vi "rszvl_core_global.vi"() -> ()   [LabVIEW 2014] (continued)
, "Flags"={"OPC Wait"=FALSE, "Dont check status"=FALSE, "*WAI"=FALSE}, "Check Status Callback"=""}, {"Level"=3, "Descriptive Name"="Delta Marker Mode", "Class Only"=FALSE, "Data Type"=0, "Access"=2, "Identifier"="RSZVL_ATTR_REFERENCE_MARKER_MODE", "Range Table"="rszvl_rngAbsRel", "Command"="CALC:DELT{DeltaMarker}:MODE", "Read Callback"="", "Write Callback"="", "Range Callback"="", "Check Callback"="", "Rngtable Callback"="", "Coerce Callback"="", "User Callback"="", "Supported Models"="", "Instrument Options"="", "Repeated Capabilities"="", "Restricted Repeated Capabilities"="", "Help"="This attribute switches between relative and absolute frequency input of the delta marker (or time with span = 0). It affects all delta markers.\nRepeated capabilitiy Delta Marker are used to prevent switching On Delta Marker 1, if the user uses Delta Marker 2.\n\nAvailable Repeated Capabilities:\nDeltaMarker: DM1,DM2,DM3,DM4\r\n\nRemote-control command(s):\nCALCulate<1|2>:DELTamarker<1 to 4>:MODE ABSolute | RELative", "Flags"={"OPC Wait"=FALSE, "Dont check status"=FALSE, "*WAI"=FALSE}, "Check Status Callback"=""}, {"Level"=3, "Descriptive Name"="Delta Marker Position", "Class Only"=FALSE, "Data Type"=1, "Access"=2, "Identifier"="RSZVL_ATTR_REFERENCE_MARKER_POSITION", "Range Table"="", "Command"="CALC:DELT{DeltaMarker}:X", "Read Callback"="", "Write Callback"="", "Range Callback"="", "Check Callback"="", "Rngtable Callback"="", "Coerce Callback"="", "User Callback"="", "Supported Models"="", "Instrument Options"="", "Repeated Capabilities"="", "Restricted Repeated Capabilities"="", "Help"="This attribute positions the selected delta marker to the indicated frequency (span > 0), time (span = 0) or level (APD measurement = ON or CCDFmeasurement = ON). The input is in absolute values or relative to marker 1 depending on the attribute RSZVL_ATTR_REFERENCE_MARKER_MODE. If Reference Fixed measurement (CALCulate:DELTamarker:FUNCtion:FIXed:STATe ON) is active, relative values refer to the reference position are entered. The query always returns absolute values.\n\nAvailable Repeated Capabilities:\nDeltaMarker: DM1,DM2,DM3,DM4\r\n\nRemote-control command(s):\nCALCulate<1|2>:DELTamarker<1 to 4>:X", "Flags"={"OPC Wait"=FALSE, "Dont check status"=FALSE, "*WAI"=FALSE}, "Check Status Callback"=""}, {"Level"=3, "Descriptive Name"="Delta Marker Relative Position", "Class Only"=FALSE, "Data Type"=1, "Access"=0, "Identifier"="RSZVL_ATTR_REFERENCE_MARKER_REL_POSITION", "Range Table"="", "Command"="CALC:DELT{DeltaMarker}:X:REL?", "Read Callback"="", "Write Callback"="", "Range Callback"="", "Check Callback"="", "Rngtable Callback"="", "Coerce Callback"="", "User Callback"="", "Supported Models"="", "Instrument Options"="", "Repeated Capabilities"="", "Restricted Repeated Capabilities"="", "Help"="This attribute queries the frequency (span > 0) or time (span = 0) of the selected delta marker relative to marker 1 or to the reference position ( for CALCulate:DELTamarker:FUNCtion:FIXed:STATe ON). The attribute activates the corresponding delta marker, if necessary.\n\nAvailable Repeated Capabilities:\nDeltaMarker: DM1,DM2,DM3,DM4\r\n\nRemote-control command(s):\nCALCulate<1|2>:DELTamarker<1 to 4>:X:RELative?", "Flags"={"OPC Wait"=FALSE, "Dont check status"=FALSE, "*WAI"=FALSE}, "Check Status Callback"=""}, {"Level"=3, "Descriptive Name"="Delta Marker Amplitude", "Class Only"=FALSE, "Data Type"=1, "Access"=0, "Identifier"="RSZVL_ATTR_REFERENCE_MARKER_AMPLITUDE", "Range Table"="", "Command"="CALC:DELT{DeltaMarker}:Y?", "Read Callback"="", "Write Callback"="", "Range Callback"="", "Check Callback"="", "Rngtable Callback"="", "Coerce Callback"="", "User Callback"="", "Supported Models"="", "Instrument Options"="", "Repeated Capabilities"="", "Restricted Repeated Capabilities"="", "Help"="This attribute queries the measured value of the selected delta marker. The corresponding delta marker will be activated, if necessary. The output is always a relative value referred to marker 1 or to the reference position (reference fixed active).\n\nAvailable Repeated Capabilities:\nDeltaMarker: DM1,DM2,DM3,DM4\r\n\nRemote-control command(s):\nCALCulate<1|2>:DELTamarker<1 to 4>:Y?", "Flags"={"OPC Wait"=FALSE, "Dont check status"=FALSE, "*WAI"=FALSE}, "Check Status Callback"=""}, {"Level"=3, "Descriptive Name"="Delta Marker Assign Trace", "Class Only"=FALSE, "Data Type"=0, "Access"=2, "Identifier"="RSZVL_ATTR_REFERENCE_MARKER_TRACE", "Range Table"="rszvl_rngTrace", "Command"="CALC:DELT{DeltaMarker}:TRAC", "Read Callback"="", "Write Callback"="", "Range Callback"="", "Check Callback"="", "Rngtable Callback"="", "Coerce Callback"="", "User Callback"="", "Supported Models"="", "Instrument Options"="", "Repeated Capabilities"="", "Restricted Repeated Capabilities"="", "Help"="This attribute assigns the selected delta marker to the indicated measurement curve. The selected measurement curve must be active, i.e. its state must be different from BLANK.\n\nAvailable Repeated Capabilities:\nDeltaMarker: DM1,DM2,DM3,DM4\r\n\nRemote-control command(s):\nCALCulate<1|2>:DELTamarker<1 to 4>:TRACe", "Flags"={"OPC Wait"=FALSE, "Dont check status"=FALSE, "*WAI"=FALSE}, "Check Status Callback"=""}, {"Level"=3, "Descriptive Name"="Delta Marker All Off", "Class Only"=FALSE, "Data Type"=4, "Access"=1, "Identifier"="RSZVL_ATTR_REFERENCE_MARKER_AOFF", "Range Table"="", "Command"="CALC:DELT:AOFF", "Read Callback"="", "Write Callback"="", "Range Callback"="", "Check Callback"="", "Rngtable Callback"="", "Coerce Callback"="", "User Callback"="", "Supported Models"="", "Instrument Options"="", "Repeated Capabilities"="", "Restricted Repeated Capabilities"="", "Help"="This attribute switches off all active delta markers (screen A or screen B).\n\nAvailable Repeated Capabilities:\nNone\n\nRemote-control command(s):\nCALCulate<1|2>:DELTamarker<1 to 4>:AOFF", "Flags"={"OPC Wait"=FALSE, "Dont check status"=FALSE, "*WAI"=FALSE}, "Check Status Callback"=""}, {"Level"=2, "Descriptive Name"="Delta Marker Search", "Class Only"=TRUE, "Data Type"=0, "Access"=0, "Identifier"="", "Range Table"="", "Command"="", "Read Callback"="", "Write Callback"="", "Range Callback"="", "Check Callback"="", "Rngtable Callback"="", "Coerce Callback"="", "User Callback"="", "Supported Models"="", "Instrument Options"="", "Repeated Capabilities"="", "Restricted Repeated Capabilities"="", "Help"="Delta marker search.\n\n(1) Delta Marker Peak:\nThis attribute positions the delta marker to the current maximum value on the measured curve. If necessary, the corresponding delta marker will be activated first.\n\n(2) Delta Marker Peak Next:\nThis attribute positions the delta marker to the next smaller maximum value on the measured curve. The corresponding delta marker will be activated first, if necessary.\n\n(3) Delta Marker Peak Next Right:\nThis attribute positions the delta marker to the next smaller maximum value to the right of the current value (i.e. ascending X values). The corresponding delta marker is activated first, if necessary.\n\n(4) Delta Marker Peak Next Left:\nThis attribute positions the delta marker to the next smaller maximum value to the left of the current value (i.e. descending X values). The corresponding delta marker will be activated first, if necessary.\n\n(5) Delta Marker Minimum:\nThis attribute positions the delta marker to the current minimum value on the measured crve. The corresponding delta marker will be activated first, if necessary.\n\n(6) Delta Marker Minimum Next:\nThis attribute positions the delta marker to the next higher minimum value of the measured curve. The corresponding delta marker will be activated first, if necessary.\n\n(7) Delta Marker Minimum Next Right:\nThis attribute positions the delta marker to the next higher minimum value to the right of the current value (i.e. ascending X values). The corresponding delta marker will be activated first, if necessary.\n\n(8) Delta Marker Minimum Next Left:\nThis attribute positions the delta marker to the next higher minimum value to the left of the current value (i.e. descending X values). The corresponding delta marker will be activated first, if necessary.", "Flags"={"OPC Wait"=FALSE, "Dont check status"=FALSE, "*WAI"=FALSE}, "Check Status Callback"=""}, {"Level"=3, "Descriptive Name"="Delta Marker Peak", "Class Only"=FALSE, "Data Type"=4, "Access"=1, "Identifier"="RSZVL_ATTR_REFERENCE_MARKER_PEAK", "Range Table"="", "Command"="CALC:DELT{DeltaMarker}:MAX", "Read Callback"="", "Write Callback"="", "Range Callback"="", "Check Callback"="", "Rngtable Callback"="", "Coerce Callback"="", "User Callback"="", "Supported Models"="", "Instrument Options"="", "Repeated Capabilities"="", "Restricted Repeated Capabilities"="", "Help"="This attribute positions the delta marker to the current maximum value on the measured curve. If necessary, the corresponding delta marker will be activated first.\n\nAvailable Repeated Capabilities:\nDeltaMarker: DM1,DM2,DM3,DM4\r\n\nRemote-control command(s):\nCALCulate<1|2>:DELTamarker<1 to 4>:MAXimum[:PEAK]", "Flags"={"OPC Wait"=FALSE, "Dont check status"=FALSE, "*WAI"=FALSE}, "Check Status Callback"=""}, {"Level"=3, "Descriptive Name"="Delta Marker Peak Next", "Class Only"=FALSE, "Data Type"=4, "Access"=1, "Identifier"="RSZVL_ATTR_REFERENCE_MARKER_PEAK_NEXT", "Range Table"="", "Command"="CALC:DELT{DeltaMarker}:MAX:NEXT", "Read Callback"="", "Write Callback"="", "Range Callback"="", "Check Callback"="", "Rngtable Callback"="", "Coerce Callback"="", "User Callback"="", "Supported Models"="", "Instrument Options"="", "Repeated Capabilities"="", "Restricted Repeated Capabilities"="", "Help"="This attribute positions the delta marker to the next smaller maximum value on the measured curve. The corresponding delta marker will be activated first, if necessary.\n\nAvailable Repeated Capabilities:\nDeltaMarker: DM1,DM2,DM3,DM4\r\n\nRemote-control command(s):\nCALCulate<1|2>:DELTamarker<1 to 4>:MAXimum:NEXT", "Flags"={"OPC Wait"=FALSE, "Dont check status"=FALSE, "*WAI"=FALSE}, "Check Status Callback"=""}, {"Level"=3, "Descriptive Name"="Delta Marker Peak Next Right", "Class Only"=FALSE, "Data Type"=4, "Access"=1, "Identifier"="RSZVL_ATTR_REFERENCE_MARKER_PEAK_NEXT_RIGHT", "Range Table"="", "Command"="CALC:DELT{DeltaMarker}:MAX:RIGH", "Read Callback"="", "Write Callback"="", "Range Callback"="", "Check Callback"="", "Rngtable Callback"="", "Coerce Callback"="", "User Callback"="", "Supported Models"="", "Instrument Options"="", "Repeated Capabilities"="", "Restricted Repeated Capabilities"="", "Help"="This attribute positions the delta marker to the next smaller maximum value to the right of the current value (i.e. ascending X values). The corresponding delta marker is activated first, if necessary.\n\nAvailable Repeated Capabilities:\nDeltaMarker: DM1,DM2,DM3,DM4\r\n\nRemote-control command(s):\nCALCulate<1|2>:DELTamarker<1 to 4>:MAXimum:RIGHt", "Flags"={"OPC Wait"=FALSE, "Dont check status"=FALSE, "*WAI"=FALSE}, "Check Status Callback"=""}, {"Level"=3, "Descriptive Name"="Delta Marker Peak Next Left", "Class Only"=FALSE, "Data Type"=4, "Access"=1, "Identifier"="RSZVL_ATTR_REFERENCE_MARKER_PEAK_NEXT_LEFT", "Range Table"="", "Command"="CALC:DELT{DeltaMarker}:MAXimum:LEFT", "Read Callback"="", "Write Callback"="", "Range Callback"="", "Check Callback"="", "Rngtable Callback"="", "Coerce Callback"="", "User Callback"="", "Supported Models"="", "Instrument Options"="", "Repeated Capabilities"="", "Restricted Repeated Capabilities"="", "Help"="This attribute positions the delta marker to the next smaller maximum value to the left of the current value (i.e. descending X values). The corresponding delta marker will be activated first, if necessary.\n\nAvailable Repeated Capabilities:\nDeltaMarker: DM1,DM2,DM3,DM4\r\n\nRemote-control command(s):\nCALCulate<1|2>:DELTamarker<1 to 4>:MAXimum:LEFT", "Flags"={"OPC Wait"=FALSE, "Dont check status"=FALSE, "*WAI"=FALSE}, "Check Status Callback"=""}, {"Level"=3, "Descriptive Name"="Delta Marker Minimum", "Class Only"=FALSE, "Data Type"=4, "Access"=1, "Identifier"="RSZVL_ATTR_REFERENCE_MARKER_MIN", "Range Table"="", "Command"="CALC:DELT{DeltaMarker}:MIN", "Read Callback"="", "Write Callback"="", "Range Callback"="", "Check Callback"="", "Rngtable Callback"="", "Coerce Callback"="", "User Callback"="", "Supported Models"="", "Instrument Options"="", "Repeated Capabilities"="", "Restricted Repeated Capabilities"="", "Help"="This attribute positions the delta marker to the current minimum value on the measured crve. The corresponding delta marker will be activated first, if necessary.\n\nAvailable Repeated Capabilities:\nDeltaMarker: DM1,DM2,DM3,DM4\r\n\nRemote-control command(s):\nCALCulate<1|2>:DELTamarker<1 to 4>:MINimum[:PEAK]", "Flags"={"OPC Wait"=FALSE, "Dont check status"=FALSE, "*WAI"=FALSE}, "Check Status Callback"=""}, {"Level"=3, "Descriptive Name"="Delta Marker Minimum Next", "Class Only"=FALSE, "Data Type"=4, "Access"=1, "Identifier"="RSZVL_ATTR_REFERENCE_MARKER_MIN_NEXT", "Range Table"="", "Command"="CALC:DELT{DeltaMarker}:MIN:NEXT", "Read Callback"="", "Write Callback"="", "Range Callback"="", "Check Callback"="", "Rngtable Callback"="", "Coerce Callback"="", "User Callback"="", "Supported Models"="", "Instrument Options"="", "Repeated Capabilities"="", "Restricted Repeated Capabilities"="", "Help"="This attribute positions the delta marker to the next higher minimum value of the measured curve. The corresponding delta marker will be activated first, if necessary.\n\nAvailable Repeated Capabilities:\nDeltaMarker: DM1,DM2,DM3,DM4\r\n\nRemote-control command(s):\nCALCulate<1|2>:DELTamarker<1 to 4>:MINimum:NEXT", "Flags"={"OPC Wait"=FALSE, "Dont check status"=FALSE, "*WAI"=FALSE}, "Check Status Callback"=""}, {"Level"=3, "Descriptive Name"="Delta Marker Minimum Next Right", "Class Only"=FALSE, "Data Type"=4, "Access"=1, "Identifier"="RSZVL_ATTR_REFERENCE_MARKER_MIN_NEXT_RIGHT", "Range Table"="", "Command"="CALC:DELT{DeltaMarker}:MIN:RIGH", "Read Callback"="", "Write Callback"="", "Range Callback"="", "Check Callback"="", "Rngtable Callback"="", "Coerce Callback"="", "User Callback"="", "Supported Models"="", "Instrument Options"="", "Repeated Capabilities"="", "Restricted Repeated Capabilities"="", "Help"="This attribute positions the delta marker to the next higher minimum value to the right of the current value (i.e. ascending X values). The corresponding delta marker will be activated first, if necessary.\n\nAvailable Repeated Capabilities:\nDeltaMarker: DM1,DM2,DM3,DM4\r\n\nRemote-control command(s):\nCALCulate<1|2>:DELTamarker<1 to 4>:MINimum:RIGHt", "Flags"={"OPC Wait"=FALSE, "Dont check status"=FALSE, "*WAI"=FALSE}, "Check Status Callback"=""}, {"Level"=3, "Descriptive Name"="Delta Marker Minimum Next Left", "Class Only"=FALSE, "Data Type"=4, "Access"=1, "Identifier"="RSZVL_ATTR_REFERENCE_MARKER_MIN_NEXT_LEFT", "Range Table"="", "Command"="CALC:DELT{DeltaMarker}:MIN:LEFT", "Read Callback"="", "Write Callback"="", "Range Callback"="", "Check Callback"="", "Rngtable Callback"="", "Coerce Callback"="", "User Callback"="", "Supported Models"="", "Instrument Options"="", "Repeated Capabilities"="", "Restricted Repeated Capabilities"="", "Help"="This attribute positions the delta marker to the next higher minimum value to the left of the current value (i.e. descending X values). The corresponding delta marker will be activated first, if necessary.\n\nAvailable Repeated Capabilities:\nDeltaMarker: DM1,DM2,DM3,DM4\r\n\nRemote-control command(s):\nCALCulate<1|2>:DELTamarker<1 to 4>:MINimum:LEFT", "Flags"={"OPC Wait"=FALSE, "Dont check status"=FALSE, "*WAI"=FALSE}, "Check Status Callback"=""}, {"Level"=1, "Descriptive Name"="Limit Lines", "Class Only"=TRUE, "Data Type"=0, "Access"=0, "Identifier"="", "Range Table"="", "Command"="", "Read Callback"="", "Write Callback"="", "Range Callback"="", "Check Callback"="", "Rngtable Callback"="", "Coerce Callback"="", "User Callback"="", "Supported Models"="", "Instrument Options"="", "Repeated Capabilities"="", "Restricted Repeated Capabilities"="", "Help"="(1) Limit Check State:\nThis attribute switches on or off the limit check for the selected limit line.\n\n(2) Limit Check Clear:\nThis attribute deletes the result of the current limit check for all limit lines.\n\n(3) Limit Line Assign Trace:\nThis attribute assigns a limit line to a trace.\n\n(4) Limit Line Units:\nThis attribute defines the unit of the selected limit line.\nUpon selection of the unit DB the limit line is automatically switched to the relative mode. For units different from DB the limit line is  automatically switched to absolute mode.\nThe units DEG, RAD, S, HZ, PCT are not available in SPECTRUM mode.\n\n(5) Limit Line Comment:\nThis attribute defines a comment for the limit line selected (max. 40 characters).\n\n(6) Limit Line Copy:\nThis attribute copies one limit line onto another one.\n\n(7) Limit Line Name:\nThis attribute assigns a name to a limit line numbered 1 to 8. If it does not exist already, a limit line with this name is created.\nThe name of the limit line may contain a maximum of 8 characters.\n\n(8) Limit Line Delete:\nThis attribute deletes the selected limit line.\n\n(9) X-Axis (Class):\n(1) Limit Line Control Domain:\nThis attribute defines the frequency or time domain for the x axis values.\n\n(2) Limit Line Control Spacing:\nThis attribute selects linear or logarithmic interpolation for the calculation of limit lines from frequency points.\n\n(3) Limit Line Control Scaling:\nThis attribute selects the relative or absolute scaling for the X axis of the selected limit line.\n\n(4) Limit Line Control Offset:\nThis attribute defines an offset for the X axis value of the selected relative limit line in the frequency or time domain.\n\n(5) Limit Line Control Shift:\nThis attribute moves a limit line by the indicated value in x direction. In contrast to offset, the line is shifted by modifying the individual x values and not by means of an additive offset.\n\n\n\n(10) Lower Limit (Class):\n(1) Limit Line Lower State:\nThis attribute switches on or off the indicated limit line.\n\n(2) Limit Line Lower Scaling:\nThis attribute selects the relative or absolute scaling for the Y axis of the selected lower limit line. Selecting RELative causes the unit to be switched to DB.\n\n(3) Limit Line Lower Spacing:\nThis attribute selects linear or logarithmic interpolation for the lower limit line.\n\n(4) Limit Line Lower Margin:\nThis attribute defines a margin to a lower limit line, at which out-of-limit values are signalled (if the limit check is active), but not handled as a violation of the limit value.\n\n(5) Limit Line Lower Threshold:\nThis attribute defines an absolute threshold value for limit lines with relative Y axis scaling. The absolute threshold value is used in the limit check as soon as it exceeds the relative limit value.\n\n(6) Limit Line Lower Offset:\nThis attribute defines an offset for the Y axis of the selected relative lower limit line. In contrast to SHIF, the line is not shifted by modifying the individual Y values but by means of an additive offset.\n\n(7) Limit Line Lower Shift:\nThis attribute shifts a limit line by the indicated value in Y direction. In contrast to offset, the line is shifted by modifying the individual Y values but not by means of an additive offset.\n\n\n\n(11) Upper Limit (Class):\n(1) Limit Line Upper State:\nThis attribute switches on or off the indicated limit line.\n\n(2) Limit Line Upper Scaling:\nThis command selects the relative or absolute scaling for the Y axis of the selected upper limit line. Selecting RELative causes the unit to be switched to DB.\n\n(3) Limit Line Upper Spacing:\nThis attribute selects linear or logarithmic interpolation for the upper limit line.\n\n(4) Limit Line Upper Margin:\nThis attribute defines a margin to an upper limit line, at which out-of-limit values are signalled (if the limit check is active), but not handled as a violation of the limit value.\n\n(5) Limit Line Upper Threshold:\nThis attribute defines an absolute threshold value for limit lines with relative Y axis scaling. The absolute threshold value is used in the limit check as soon as it exceeds the relative limit value.\n\n(6) Limit Line Upper Offset:\nThis attribute defines an offset for the Y axis of the selected relative upper limit line. In contrast to shift, the line is not shifted by modifying the individual Y values but by means of an additive offset.\n\n(7) Limit Line Upper Shift:\nThis attribute moves a limit line by the indicated value in Y direction. In contrast to offset, the line is shifted by modifying the individual Y values and not by means of an additive offset.\n\n\n\n(12) Display Lines (Class):\n(1) Threshold Line State:\nThis attribute switches on or off the threshold line.\n\n(2) Threshold Line Position:\nThis attribute defines the threshold value for the maximum/minimum search of markers with marker search functions MAX PEAK, NEXT PEAK, etc.\n\n(3) Display Line State:\nThis attribute switches Display Line 1 or 2 (level lines) on or off.\n\n(4) Display Line Position:\nThis attribute defines the position of Display Line 1 or 2. These lines enable the user to mark any levels in the diagram. The unit depends on the setting made with CALC:UNIT.\n\n(5) Frequency Line State:\nThis attribute switches the frequency line on or off.\n\n(6) Frequency Line Position:\nThis attribute defines the position of the frequency lines.\nThe frequency lines mark the frequencies. Frequency lines are only available with SPAN > 0.\n\n(7) Time Line State:\nThis attribute switches the time line on or off.\n\n(8) Time Line Position:\nThis attribute defines the position of the time lines.\nThe time lines mark the times. Time lines are only available with SPAN = 0.", "Flags"={"OPC Wait"=FALSE, "Dont check status"=FALSE, "*WAI"=FALSE}, "Check Status Callback"=""}, {"Level"=2, "Descriptive Name"="Limit Check State", "Class Only"=FALSE, "Data Type"=3, "Access"=2, "Identifier"="RSZVL_LIMIT_STATE", "Range Table"="", "Command"="CALC:LIM{Limit}:STAT", "Read Callback"="", "Write Callback"="", "Range Callback"="", "Check Callback"="", "Rngtable Callback"="", "Coerce Callback"="", "User Callback"="", "Supported Models"="", "Instrument Options"="", "Repeated Capabilities"="", "Restricted Repeated Capabilities"="", "Help"="This attribute switches on or off the limit check for the selected limit line.\n\nAvailable Repeated Capabilities:\nLimit: L1,L2,L3,L4,L5,L6,L7,L8\r\n\nRemote-control command(s):\nCALCulate<1|2>:LIMit<1 to 8>:STATe ON | OFF", "Flags"={"OPC Wait"=FALSE, "Dont check status"=FALSE, "*WAI"=FALSE}, "Check Status Callback"=""}, {"Level"=2, "Descriptive Name"="Limit Check Clear", "Class Only"=FALSE, "Data Type"=4, "Access"=1, "Identifier"="RSZVL_LIMIT_CLEAR", "Range Table"="", "Command"="CALC:LIM{Limit}:CLE", "Read Callback"="", "Write Callback"="", "Range Callback"="", "Check Callback"="", "Rngtable Callback"="", "Coerce Callback"="", "User Callback"="", "Supported Models"="", "Instrument Options"="", "Repeated Capabilities"="", "Restricted Repeated Capabilities"="", "Help"="This attribute deletes the result of the current limit check for all limit lines.\n\nAvailable Repeated Capabilities:\nLimit: L1,L2,L3,L4,L5,L6,L7,L8\r\n\nRemote-control command(s):\nCALCulate<1|2>:LIMit<1 to 8>:CLEar[:IMMediate]", "Flags"={"OPC Wait"=FALSE, "Dont check status"=FALSE, "*WAI"=FALSE}, "Check Status Callback"=""}, {"Level"=2, "Descriptive Name"="Limit Line Assign Trace", "Class Only"=FALSE, "Data Type"=0, "Access"=2, "Identifier"="RSZVL_LIMIT_ASSIGN_TRACE", "Range Table"="rszvl_rngTrace", "Command"="CALC:LIM{Limit}:TRAC", "Read Callback"="", "Write Callback"="", "Range Callback"="", "Check Callback"="", "Rngtable Callback"="", "Coerce Callback"="", "User Callback"="", "Supported Models"="", "Instrument Options"="", "Repeated Capabilities"="", "Restricted Repeated Capabilities"="", "Help"="This attribute assigns a limit line to a trace.\n\nAvailable Repeated Capabilities:\nLimit: L1,L2,L3,L4,L5,L6,L7,L8\r\n\nRemote-control command(s):\nCALCulate<1|2>:LIMit<1 to 8>:TRACe", "Flags"={"OPC Wait"=FALSE, "Dont check status"=FALSE, "*WAI"=FALSE}, "Check Status Callback"=""}, {"Level"=2, "Descriptive Name"="Limit Line Units", "Class Only"=FALSE, "Data Type"=0, "Access"=2, "Identifier"="RSZVL_LIMIT_UNITS", "Range Table"="rszvl_rngUnits", "Command"="CALC:LIM{Limit}:UNIT", "Read Callback"="", "Write Callback"="", "Range Callback"="", "Check Callback"="", "Rngtable Callback"="", "Coerce Callback"="", "User Callback"="", "Supported Models"="", "Instrument Options"="", "Repeated Capabilities"="", "Restricted Repeated Capabilities"="", "Help"="This attribute defines the unit of the selected limit line.\nUpon selection of the unit DB the limit line is automatically switched to the relative mode. For units different from DB the limit line is  automatically switched to absolute mode.\nThe units DEG, RAD, S, HZ, PCT are not available in SPECTRUM mode.\n\nAvailable Repeated Capabilities:\nLimit: L1,L2,L3,L4,L5,L6,L7,L8\r\n\nRemote-control command(s):\nCALCulate<1|2>:LIMit<1 to 8>:UNIT", "Flags"={"OPC Wait"=FALSE, "Dont check status"=FALSE, "*WAI"=FALSE}, "Check Status Callback"=""}, {"Level"=2, "Descriptive Name"="Limit Line Comment", "Class Only"=FALSE, "Data Type"=2, "Access"=2, "Identifier"="RSZVL_LIMIT_COMMENT", "Range Table"="", "Command"="CALC:LIM{Limit}:COMM", "Read Callback"="rszvl_quotedString_ReadCallback.vi", "Write Callback"="rszvl_quotedString_WriteCallback.vi", "Range Callback"="", "Check Callback"="", "Rngtable Callback"="", "Coerce Callback"="", "User Callback"="", "Supported Models"="", "Instrument Options"="", "Repeated Capabilities"="", "Restricted Repeated Capabilities"="", "Help"="This attribute defines a comment for the limit line selected (max. 40 characters).\n\nAvailable Repeated Capabilities:\nLimit: L1,L2,L3,L4,L5,L6,L7,L8\r\n\nRemote-control command(s):\nCALCulate<1|2>:LIMit<1 to 8>:COMMent", "Flags"={"OPC Wait"=FALSE, "Dont check status"=FALSE, "*WAI"=FALSE}, "Check Status Callback"=""}, {"Level"=2, "Descriptive Name"="Limit Line Copy", "Class Only"=FALSE, "Data Type"=0, "Access"=1, "Identifier"="RSZVL_LIMIT_COPY", "Range Table"="rszvl_rngLimits", "Command"="CALC:LIM{Limit}:COPY", "Read Callback"="", "Write Callback"="", "Range Callback"="", "Check Callback"="", "Rngtable Callback"="", "Coerce Callback"="", "User Callback"="", "Supported Models"="", "Instrument Options"="", "Repeated Capabilities"="", "Restricted Repeated Capabilities"="", "Help"="This attribute copies one limit line onto another one.\n\nAvailable Repeated Capabilities:\nLimit: L1,L2,L3,L4,L5,L6,L7,L8\r\n\nRemote-control command(s):\nCALCulate<1|2>:LIMit<1 to 8>:COPY", "Flags"={"OPC Wait"=FALSE, "Dont check status"=FALSE, "*WAI"=FALSE}, "Check Status Callback"=""}, {"Level"=2, "Descriptive Name"="Limit Line Name", "Class Only"=FALSE, "Data Type"=2, "Access"=2, "Identifier"="RSZVL_LIMIT_NAME", "Range Table"="", "Command"="CALC:LIM{Limit}:NAME", "Read Callback"="rszvl_quotedString_ReadCallback.vi", "Write Callback"="rszvl_quotedString_WriteCallback.vi", "Range Callback"="", "Check Callback"="", "Rngtable Callback"="", "Coerce Callback"="", "User Callback"="", "Supported Models"="", "Instrument Options"="", "Repeated Capabilities"="", "Restricted Repeated Capabilities"="", "Help"="This attribute assigns a name to a limit line numbered 1 to 8. If it does not exist already, a limit line with this name is created.\nThe name of the limit line may contain a maximum of 8 characters.\n\nAvailable Repeated Capabilities:\nLimit: L1,L2,L3,L4,L5,L6,L7,L8\r\n\nRemote-control command(s):\nCALCulate<1|2>:LIMit<1 to 8>:NAME", "Flags"={"OPC Wait"=FALSE, "Dont check status"=FALSE, "*WAI"=FALSE}, "Check Status Callback"=""}, {"Level"=2, "Descriptive Name"="Limit Line Delete", "Class Only"=FALSE, "Data Type"=4, "Access"=1, "Identifier"="RSZVL_LIMIT_DELETE", "Range Table"="", "Command"="CALC:LIM{Limit}:DELete", "Read Callback"="", "Write Callback"="", "Range Callback"="", "Check Callback"="", "Rngtable Callback"="", "Coerce Callback"="", "User Callback"="", "Supported Models"="", "Instrument Options"="", "Repeated Capabilities"="", "Restricted Repeated Capabilities"="", "Help"="This attribute deletes the selected limit line.\n\nAvailable Repeated Capabilities:\nLimit: L1,L2,L3,L4,L5,L6,L7,L8\r\n\nRemote-control command(s):\nCALCulate<1|2>:LIMit<1 to 8>:DELete", "Flags"={"OPC Wait"=FALSE, "Dont check status"=FALSE, "*WAI"=FALSE}, "Check Status Callback"=""}, {"Level"=2, "Descriptive Name"="X-Axis", "Class Only"=TRUE, "Data Type"=0, "Access"=0, "Identifier"="", "Range Table"="", "Command"="", "Read Callback"="", "Write Callback"="", "Range Callback"="", "Check Callback"="", "Rngtable Callback"="", "Coerce Callback"="", "User Callback"="", "Supported Models"="", "Instrument Options"="", "Repeated Capabilities"="", "Restricted Repeated Capabilities"="", "Help"="(1) Limit Line Control Domain:\nThis attribute defines the frequency or time domain for the x axis values.\n\n(2) Limit Line Control Spacing:\nThis attribute selects linear or logarithmic interpolation for the calculation of limit lines from frequency points.\n\n(3) Limit Line Control Scaling:\nThis attribute selects the relative or absolute scaling for the X axis of the selected limit line.\n\n(4) Limit Line Control Offset:\nThis attribute defines an offset for the X axis value of the selected relative limit line in the frequency or time domain.\n\n(5) Limit Line Control Shift:\nThis attribute moves a limit line by the indicated value in x direction. In contrast to offset, the line is shifted by modifying the individual x values and not by means of an additive offset.", "Flags"={"OPC Wait"=FALSE, "Dont check status"=FALSE, "*WAI"=FALSE}, "Check Status Callback"=""}, {"Level"=3, "Descriptive Name"="Limit Line Control Domain", "Class Only"=FALSE, "Data Type"=0, "Access"=2, "Identifier"="RSZVL_LIMIT_CONTROL_DOMAIN", "Range Table"="rszvl_rngDomain", "Command"="CALC:LIM{Limit}:CONT:DOM", "Read Callback"="", "Write Callback"="", "Range Callback"="", "Check Callback"="", "Rngtable Callback"="", "Coerce Callback"="", "User Callback"="", "Supported Models"="", "Instrument Options"="", "Repeated Capabilities"="", "Restricted Repeated Capabilities"="", "Help"="This attribute defines the frequency or time domain for the x axis values.\n\nAvailable Repeated Capabilities:\nLimit: L1,L2,L3,L4,L5,L6,L7,L8\r\n\nRemote-control command(s):\nCALCulate<1|2>:LIMit<1 to 8>:CONTrol:DOMain FREQuency | TIME", "Flags"={"OPC Wait"=FALSE, "Dont check status"=FALSE, "*WAI"=FALSE}, "Check Status Callback"=""}, {"Level"=3, "Descriptive Name"="Limit Line Control Spacing", "Class Only"=FALSE, "Data Type"=0, "Access"=2, "Identifier"="RSZVL_LIMIT_CONTROL_SPACING", "Range Table"="rszvl_rngLinLog", "Command"="CALC:LIM{Limit}:CONT:SPAC", "Read Callback"="", "Write Callback"="", "Range Callback"="", "Check Callback"="", "Rngtable Callback"="", "Coerce Callback"="", "User Callback"="", "Supported Models"="", "Instrument Options"="", "Repeated Capabilities"="", "Restricted Repeated Capabilities"="", "Help"="This attribute selects linear or logarithmic interpolation for the calculation of limit lines from frequency points.\n\nAvailable Repeated Capabilities:\nLimit: L1,L2,L3,L4,L5,L6,L7,L8\r\n\nRemote-control command(s):\nCALCulate<1|2>:LIMit<1 ... 8>:CONTrol:SPACing LINear | LOGarithmic", "Flags"={"OPC Wait"=FALSE, "Dont check status"=FALSE, "*WAI"=FALSE}, "Check Status Callback"=""}, {"Level"=3, "Descriptive Name"="Limit Line Control Scaling", "Class Only"=FALSE, "Data Type"=0, "Access"=2, "Identifier"="RSZVL_LIMIT_CONTROL_SCALING", "Range Table"="rszvl_rngAbsRel", "Command"="CALC:LIM{Limit}:CONT:MODE", "Read Callback"="", "Write Callback"="", "Range Callback"="", "Check Callback"="", "Rngtable Callback"="", "Coerce Callback"="", "User Callback"="", "Supported Models"="", "Instrument Options"="", "Repeated Capabilities"="", "Restricted Repeated Capabilities"="", "Help"="This attribute selects the relative or absolute scaling for the X axis of the selected limit line.\n\nAvailable Repeated Capabilities:\nLimit: L1,L2,L3,L4,L5,L6,L7,L8\r\n\nRemote-control command(s):\nCALCulate<1|2>:LIMit<1 to 8>:CONTrol:MODE RELative | ABSolute", "Flags"={"OPC Wait"=FALSE, "Dont check status"=FALSE, "*WAI"=FALSE}, "Check Status Callback"=""}, {"Level"=3, "Descriptive Name"="Limit Line Control Offset", "Class Only"=FALSE, "Data Type"=1, "Access"=2, "Identifier"="RSZVL_LIMIT_CONTROL_OFFSET", "Range Table"="rszvl_rngLimitOffset", "Command"="CALC:LIM{Limit}:CONT:OFFS", "Read Callback"="", "Write Callback"="", "Range Callback"="", "Check Callback"="", "Rngtable Callback"="", "Coerce Callback"="", "User Callback"="", "Supported Models"="", "Instrument Options"="", "Repeated Capabilities"="", "Restricted Repeated Capabilities"="", "Help"="This attribute defines an offset for the X axis value of the selected relative limit line in the frequency or time domain.\nThe unit of values depends on the frequency or time domain of the X axis (RSZVL_LIMIT_CONTROL_DOMAIN).\n\nAvailable Repeated Capabilities:\nLimit: L1,L2,L3,L4,L5,L6,L7,L8\r\n\nRemote-control command(s):\nCALCulate<1|2>:LIMit<1 to 8>:CONTrol:OFFSet", "Flags"={"OPC Wait"=FALSE, "Dont check status"=FALSE, "*WAI"=FALSE}, "Check Status Callback"=""}, {"Level"=3, "Descriptive Name"="Limit Line Control Shift", "Class Only"=FALSE, "Data Type"=1, "Access"=1, "Identifier"="RSZVL_LIMIT_CONTROL_SHIFT", "Range Table"="rszvl_rngLimitOffset", "Command"="CALC:LIM{Limit}:CONT:SHIF", "Read Callback"="", "Write Callback"="", "Range Callback"="", "Check Callback"="", "Rngtable Callback"="", "Coerce Callback"="", "User Callback"="", "Supported Models"="", "Instrument Options"="", "Repeated Capabilities"="", "Restricted Repeated Capabilities"="", "Help"="This attribute moves a limit line by the indicated value in x direction. In contrast to offset, the line is shifted by modifying the individual x values and not by means of an additive offset.\n\nAvailable Repeated Capabilities:\nLimit: L1,L2,L3,L4,L5,L6,L7,L8\r\n\nRemote-control command(s):\nCALCulate<1|2>:LIMit<1 to 8>:CONTrol:SHIFt", "Flags"={"OPC Wait"=FALSE, "Dont check status"=FALSE, "*WAI"=FALSE}, "Check Status Callback"=""}, {"Level"=2, "Descriptive Name"="Lower Limit", "Class Only"=TRUE, "Data Type"=0, "Access"=0, "Identifier"="", "Range Table"="", "Command"="", "Read Callback"="", "Write Callback"="", "Range Callback"="", "Check Callback"="", "Rngtable Callback"="", "Coerce Callback"="", "User Callback"="", "Supported Models"="", "Instrument Options"="", "Repeated Capabilities"="", "Restricted Repeated Capabilities"="", "Help"="(1) Limit Line Lower State:\nThis attribute switches on or off the indicated limit line.\n\n(2) Limit Line Lower Scaling:\nThis attribute selects the relative or absolute scaling for the Y axis of the selected lower limit line. Selecting RELative causes the unit to be switched to DB.\n\n(3) Limit Line Lower Spacing:\nThis attribute selects linear or logarithmic interpolation for the lower limit line.\n\n(4) Limit Line Lower Margin:\nThis attribute defines a margin to a lower limit line, at which out-of-limit values are signalled (if the limit check is active), but not handled as a violation of the limit value.\n\n(5) Limit Line Lower Threshold:\nThis attribute defines an absolute threshold value for limit lines with relative Y axis scaling. The absolute threshold value is used in the limit check as soon as it exceeds the relative limit value.\n\n(6) Limit Line Lower Offset:\nThis attribute defines an offset for the Y axis of the selected relative lower limit line. In contrast to SHIF, the line is not shifted by modifying the individual Y values but by means of an additive offset.\n\n(7) Limit Line Lower Shift:\nThis attribute shifts a limit line by the indicated value in Y direction. In contrast to offset, the line is shifted by modifying the individual Y values but not by means of an additive offset.", "Flags"={"OPC Wait"=FALSE, "Dont check status"=FALSE, "*WAI"=FALSE}, "Check Status Callback"=""}, {"Level"=3, "Descriptive Name"="Limit Line Lower State", "Class Only"=FALSE, "Data Type"=3, "Access"=2, "Identifier"="RSZVL_LIMIT_LOWER_STATE", "Range Table"="", "Command"="CALC:LIM{Limit}:LOW:STAT", "Read Callback"="", "Write Callback"="", "Range Callback"="", "Check Callback"="", "Rngtable Callback"="", "Coerce Callback"="", "User Callback"="", "Supported Models"="", "Instrument Options"="", "Repeated Capabilities"="", "Restricted Repeated Capabilities"="", "Help"="This attribute switches on or off the indicated limit line.\n\nAvailable Repeated Capabilities:\nLimit: L1,L2,L3,L4,L5,L6,L7,L8\r\n\nRemote-control command(s):\nCALCulate<1|2>:LIMit<1 to 8>:LOWer:STATe ON | OFF", "Flags"={"OPC Wait"=FALSE, "Dont check status"=FALSE, "*WAI"=FALSE}, "Check Status Callback"=""}, {"Level"=3, "Descriptive Name"="Limit Line Lower Scaling", "Class Only"=FALSE, "Data Type"=0, "Access"=2, "Identifier"="RSZVL_LIMIT_LOWER_SCALING", "Range Table"="rszvl_rngAbsRel", "Command"="CALC:LIM{Limit}:LOW:MODE", "Read Callback"="", "Write Callback"="", "Range Callback"="", "Check Callback"="", "Rngtable Callback"="", "Coerce Callback"="", "User Callback"="", "Supported Models"="", "Instrument Options"="", "Repeated Capabilities"="", "Restricted Repeated Capabilities"="", "Help"="This attribute selects the relative or absolute scaling for the Y axis of the selected lower limit line. Selecting RELative causes the unit to be switched to DB.\n\nAvailable Repeated Capabilities:\nLimit: L1,L2,L3,L4,L5,L6,L7,L8\r\n\nRemote-control command(s):\nCALCulate<1|2>:LIMit<1 to 8>:LOWer:MODE RELative | ABSolute", "Flags"={"OPC Wait"=FALSE, "Dont check status"=FALSE, "*WAI"=FALSE}, "Check Status Callback"=""}, {"Level"=3, "Descriptive Name"="Limit Line Lower Spacing", "Class Only"=FALSE, "Data Type"=0, "Access"=2, "Identifier"="RSZVL_LIMIT_LOWER_SPACING", "Range Table"="rszvl_rngLinLog", "Command"="CALC:LIM{Limit}:LOW:SPAC", "Read Callback"="", "Write Callback"="", "Range Callback"="", "Check Callback"="", "Rngtable Callback"="", "Coerce Callback"="", "User Callback"="", "Supported Models"="", "Instrument Options"="", "Repeated Capabilities"="", "Restricted Repeated Capabilities"="", "Help"="This attribute selects linear or logarithmic interpolation for the lower limit line.\n\nAvailable Repeated Capabilities:\nLimit: L1,L2,L3,L4,L5,L6,L7,L8\r\n\nRemote-control command(s):\nCALCulate<1|2>:LIMit<1 to 8>:LOWer:SPACing LINear | LOGarithmic", "Flags"={"OPC Wait"=FALSE, "Dont check status"=FALSE, "*WAI"=FALSE}, "Check Status Callback"=""}, {"Level"=3, "Descriptive Name"="Limit Line Lower Margin", "Class Only"=FALSE, "Data Type"=1, "Access"=2, "Identifier"="RSZVL_LIMIT_LOWER_MARGIN", "Range Table"="rszvl_rngLimitMargin", "Command"="CALC:LIM{Limit}:LOW:MARG", "Read Callback"="", "Write Callback"="", "Range Callback"="", "Check Callback"="", "Rngtable Callback"="", "Coerce Callback"="", "User Callback"="", "Supported Models"="", "Instrument Options"="", "Repeated Capabilities"="", "Restricted Repeated Capabilities"="", "Help"="This attribute defines a margin to a lower limit line, at which out-of-limit values are signalled (if the limit check is active), but not handled as a violation of the limit value.\n\nAvailable Repeated Capabilities:\nLimit: L1,L2,L3,L4,L5,L6,L7,L8\r\n\nRemote-control command(s):\nCALCulate<1|2>:LIMit<1 to 8>:LOWer:MARGin", "Flags"={"OPC Wait"=FALSE, "Dont check status"=FALSE, "*WAI"=FALSE}, "Check Status Callback"=""}, {"Level"=3, "Descriptive Name"="Limit Line Lower Threshold", "Class Only"=FALSE, "Data Type"=1, "Access"=2, "Identifier"="RSZVL_LIMIT_LOWER_THRESHOLD", "Range Table"="rszvl_rngRefLevel", "Command"="CALC:LIM{Limit}:LOW:THR", "Read Callback"="", "Write Callback"="", "Range Callback"="", "Check Callback"="", "Rngtable 
